vi "DrawTrajectory.vi"(0 "Image":T2, 1 "PuckCentre":cluster{sgl, sgl}, 2 "HomePoint(pixels)":cluster{dbl, dbl}, 5 "TrajectoryArray":T1, 7 "ChosenPath":i32, 9 "Pixel/mm":dbl format="%#_13g", 11 "error in (no error)":errorcluster) -> (4 "ImageOut":T2(plugin-control), 15 "error out":errorcluster)   [LabVIEW 2017]
uses:
  <vilib>/vision/Image Controls.llb/IMAQ Image.ctl
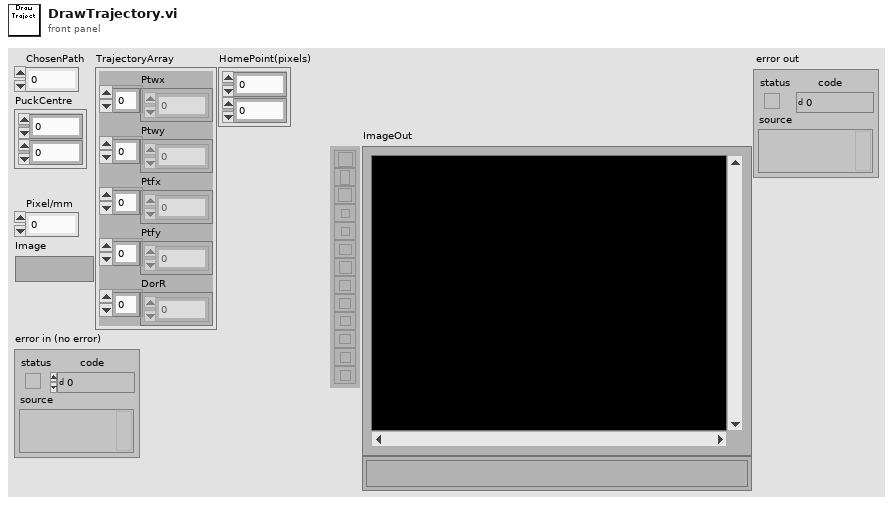
[diagram p1: front panel]
types:
  T1 = cluster{"Ptwx":dbl[], "Ptwy":dbl[], "Ptfx":dbl[], "Ptfy":dbl[], "DorR":i32[]}
  T2 = typedef "IMAQ Image.ctl" = refnum<image>
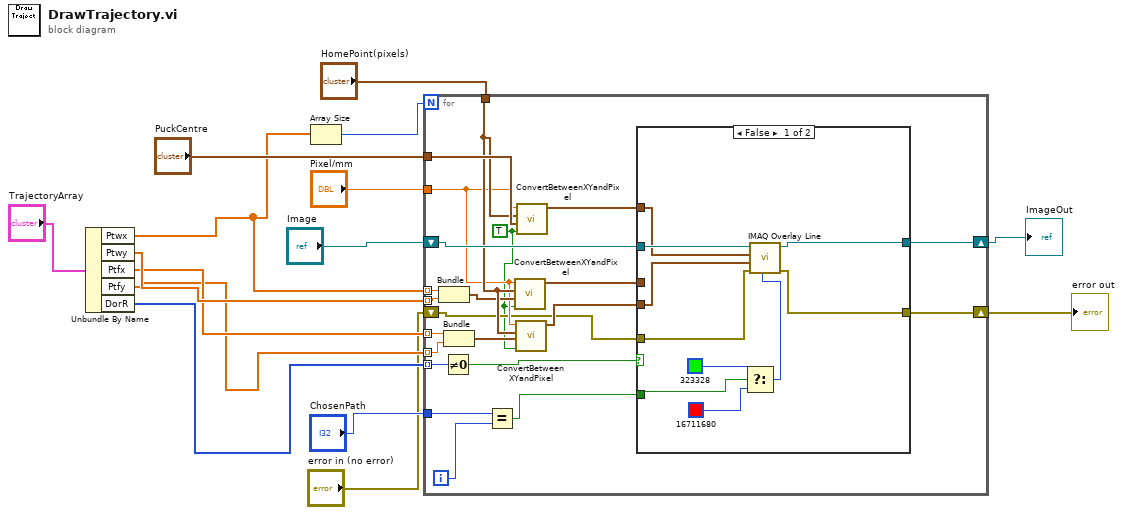
[diagram p0: block diagram]
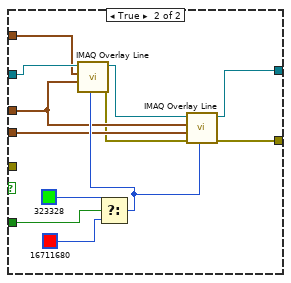
[diagram p2: hidden frame]
diagram:
  n1 = Unbundle By Name("TrajectoryArray") -> ("Ptwx"=w7:dbl[], "Ptwy"=w6:dbl[], "Ptfx"=w5:dbl[], "Ptfy"=w4:dbl[], "DorR"=w3:i32[])
  n2 = Array Size(array=w7) -> (size(s)=w14:i32)
  n3 = for {
    N: w14 -> [_]
    shift-right: [w34] -> w9
    shift-left: "Image" -> [w35]
    tunnel: w3 -> [w37] mode=indexing
    tunnel: w7 -> [w33] mode=indexing
    tunnel: w6 -> [w32] mode=indexing
    tunnel: w5 -> [w31] mode=indexing
    tunnel: w4 -> [w30] mode=indexing
    tunnel: "ChosenPath" -> [w28]
    tunnel: "HomePoint(pixels)" -> [w25]
    tunnel: "PuckCentre" -> [w26]
    tunnel: "Pixel/mm" -> [w22]
    shift-right: [w18] -> w2
    shift-left: "error in (no error)" -> [w17]
    i -> [w29]
    w16 = TRUE ("XYtoPixels")
    n4 = Bundle(w33, w32) -> (w23:cluster{dbl, dbl})  [unwired: 1 in]
    n5 = Not Equal To 0?(x=w37) -> (x != 0?=w36:bool)
    n6 = Bundle(w31, w30) -> (w24:cluster{dbl, dbl})  [unwired: 1 in]
    n7 = Equal?(x=w28, y=w29) -> (x = y?=w27:bool)
    n8 = call "ConvertBetweenXYandPixel.vi"("XYtoPixels"=w16, "PointToConvert"=w23, "HomeXY(pixels)"=w25, "Pixel/mm"=w22) -> ("Point"=w20:cluster{sgl, sgl})  [unwired: 7 in]
    n9 = call "ConvertBetweenXYandPixel.vi"("XYtoPixels"=w16, "PointToConvert"=w24, "HomeXY(pixels)"=w25, "Pixel/mm"=w22) -> ("Point"=w19:cluster{sgl, sgl})  [unwired: 7 in]
    n10 = call "ConvertBetweenXYandPixel.vi"("XYtoPixels"=w16, "PointToConvert"=w26, "HomeXY(pixels)"=w25, "Pixel/mm"=w22) -> ("Point"=w21:cluster{sgl, sgl})  [unwired: 7 in]
    n11 = case shown="False" w36 {
      tunnel: w35 -> [w47 w59]
      tunnel: [w46 w57] -> w34
      tunnel: w27 -> [w43 w56]
      tunnel: w21 -> [w41 w52]
      tunnel: w20 -> [_ w51]
      tunnel: w19 -> [w40 w50]
      tunnel: [w39 w48] -> w18
      tunnel: w17 -> [w38 _]
      frame False {
        n12 = Select(t=u32 323328 ("Color"), s=w43, f=u32 16711680 ("Color")) -> (s? t:f=w42:u32)
        n13 = call "IMAQ Overlay Line"("Color"=w42, "error in (no error)"=w38, "End Point"=w40, "Start Point"=w41, "Image"=w47) -> ("error out"=w39:errorcluster, "Image Out"=w46:T2)  [unwired: 5 in]
      }
      frame True {
        n14 = Select(t=u32 323328 ("Color"), s=w56, f=u32 16711680 ("Color")) -> (s? t:f=w53:u32)
        n15 = call "IMAQ Overlay Line"("Color"=w53, "End Point"=w51, "Start Point"=w52, "Image"=w59) -> ("error out"=w49:errorcluster, "Image Out"=w58:T2)  [unwired: 6 in]
        n16 = call "IMAQ Overlay Line"("Color"=w53, "error in (no error)"=w49, "End Point"=w50, "Start Point"=w51, "Image"=w58) -> ("error out"=w48:errorcluster, "Image Out"=w57:T2)  [unwired: 5 in]
      }
    }
  }
  "ImageOut" <- w9
  "error out" <- w2
